vi "Base64ToHexString.vi"(1 "BASE64 string":string) -> (0 "Hex":string)   [LabVIEW 2023]
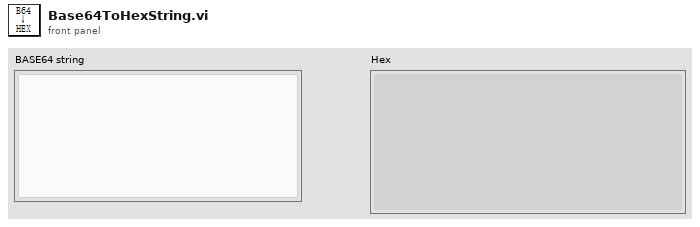
[diagram p1: front panel]
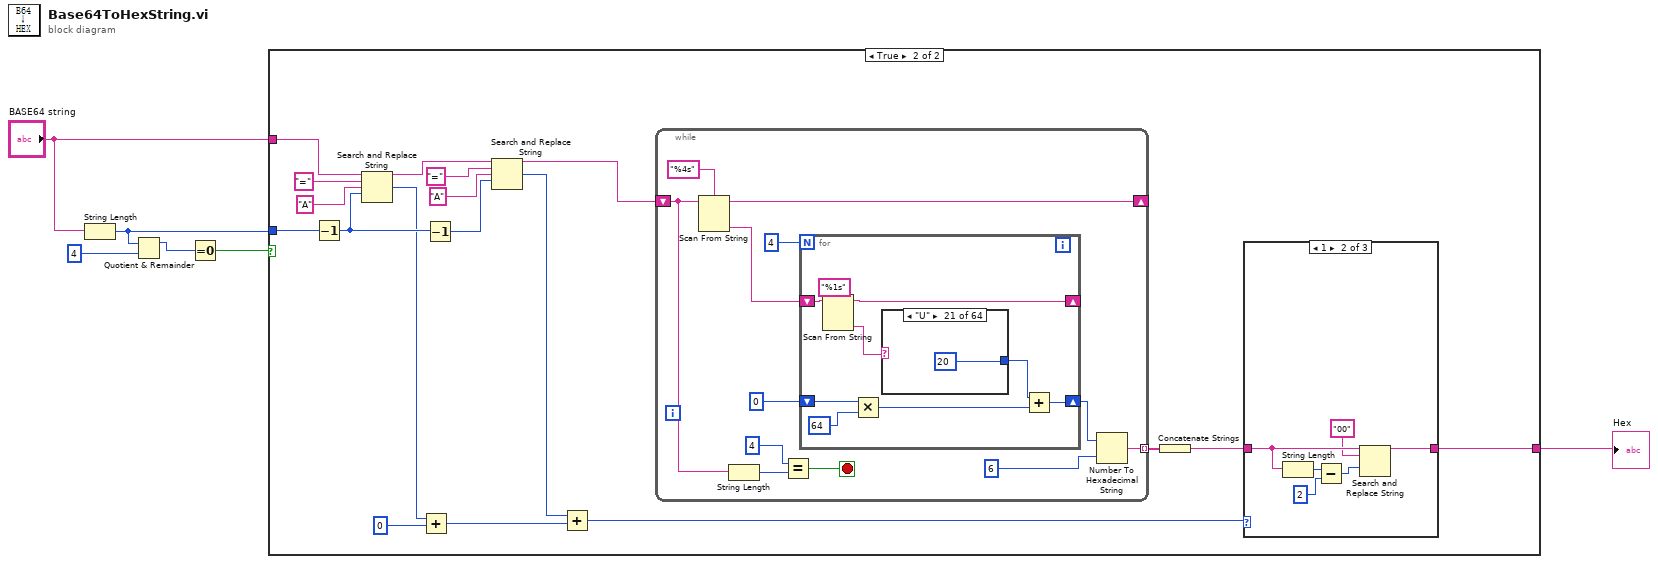
[diagram p0: block diagram]
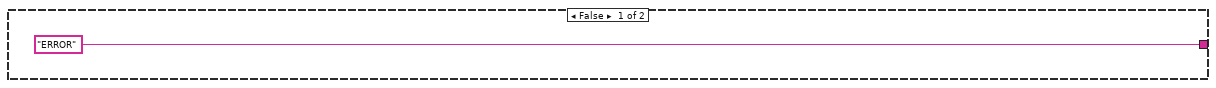
[diagram p2: hidden frame]
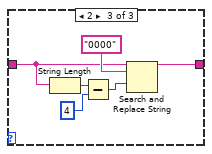
[diagram p4: hidden frame]
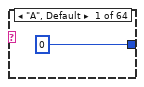
[diagram p5: hidden frame]
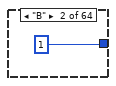
[diagram p6: hidden frame]
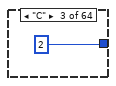
[diagram p7: hidden frame]
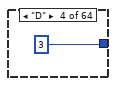
[diagram p8: hidden frame]
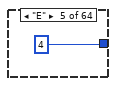
[diagram p9: hidden frame]
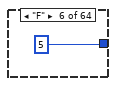
[diagram p10: hidden frame]
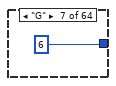
[diagram p11: hidden frame]
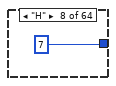
[diagram p12: hidden frame]
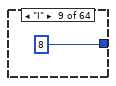
[diagram p13: hidden frame]
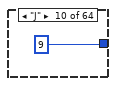
[diagram p14: hidden frame]
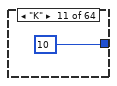
[diagram p15: hidden frame]
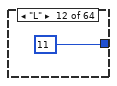
[diagram p16: hidden frame]
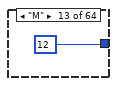
[diagram p17: hidden frame]
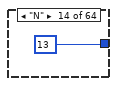
[diagram p18: hidden frame]
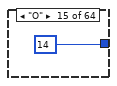
[diagram p19: hidden frame]
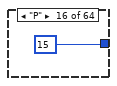
[diagram p20: hidden frame]
diagram:
  n1 = String Length(string="BASE64 string") -> (length=w4:i32)
  n2 = Quotient & Remainder(x=w4, y=4) -> (x-y*floor(x/y)=w3:i32)  [unwired: 1 out]
  n3 = Equal To 0?(x=w3) -> (x = 0?=w2:bool)
  n4 = case shown="True" w2 {
    tunnel: "BASE64 string" -> [_ w23]
    tunnel: w4 -> [_ w14]
    tunnel: ["ERROR" w8] -> w1
    frame False {
    }
    frame True {
      n5 = Decrement(x=w14) -> (x-1=w22:i32)
      n6 = Search and Replace String(input string=w23, search string="=", replace string="A", offset=w22) -> (result string=w19:string, number of replacements=w16:i32)  [unwired: 4 in, 2 out]
      n7 = Add(x=w16, y=0) -> (x+y=w17:i32)
      n8 = Decrement(x=w22) -> (x-1=w18:i32)
      n9 = Search and Replace String(input string=w19, search string="=", replace string="A", offset=w18) -> (result string=w12:string, number of replacements=w15:i32)  [unwired: 4 in, 2 out]
      n10 = Add(x=w15, y=w17) -> (x+y=w10:i32)
      n11 = while {
        shift-right: [w49] -> _
        shift-left: w12 -> [w41]
        tunnel: [w43] -> w11 mode=indexing
        stop <- w39 stop-if-true
        n12 = Scan From String(format string="%4s", input string=w41) -> (remaining string=w49:string, output 1=w48:string)  [unwired: 3 in, 2 out]
        n13 = String Length(string=w41) -> (length=w40:i32)
        n14 = Equal?(x=4, y=w40) -> (x = y?=w39:bool)
        n15 = for {
          N: 4 -> [_]
          shift-right: [w52] -> w45
          shift-left: 0 -> [w56]
          shift-right: [w51] -> _
          shift-left: w48 -> [w58]
          n16 = Scan From String(format string="%1s", input string=w58) -> (remaining string=w51:string, output 1=w57:string)  [unwired: 3 in, 2 out]
          n17 = Multiply(x=w56, y=64) -> (x*y=w54:i32)
          n18 = case shown="\"U\"" w57 {
            tunnel: [0 1 2 3 4 5 6 7 8 9 10 11 12 13 14 15 16 17 18 19 20 21 22 23 24 25 26 27 28 29 30 31 32 33 34 35 36 37 38 39 40 41 42 43 44 45 46 47 48 49 50 51 52 53 54 55 56 57 58 59 60 61 62 63] -> w53
            frame "A", Default {
            }
            frame "B" {
            }
            frame "C" {
            }
            frame "D" {
            }
            frame "E" {
            }
            frame "F" {
            }
            frame "G" {
            }
            frame "H" {
            }
            frame "I" {
            }
            frame "J" {
            }
            frame "K" {
            }
            frame "L" {
            }
            frame "M" {
            }
            frame "N" {
            }
            frame "O" {
            }
            frame "P" {
            }
            frame "Q" {
            }
            frame "R" {
            }
            frame "S" {
            }
            frame "T" {
            }
            frame "U" {
            }
            frame "V" {
            }
            frame "W" {
            }
            frame "X" {
            }
            frame "Y" {
            }
            frame "Z" {
            }
            frame "a" {
            }
            frame "b" {
            }
            frame "c" {
            }
            frame "d" {
            }
            frame "e" {
            }
            frame "f" {
            }
            frame "g" {
            }
            frame "h" {
            }
            frame "i" {
            }
            frame "j" {
            }
            frame "k" {
            }
            frame "l" {
            }
            frame "m" {
            }
            frame "n" {
            }
            frame "o" {
            }
            frame "p" {
            }
            frame "q" {
            }
            frame "r" {
            }
            frame "s" {
            }
            frame "t" {
            }
            frame "u" {
            }
            frame "v" {
            }
            frame "w" {
            }
            frame "x" {
            }
            frame "y" {
            }
            frame "z" {
            }
            frame "0" {
            }
            frame "1" {
            }
            frame "2" {
            }
            frame "3" {
            }
            frame "4" {
            }
            frame "5" {
            }
            frame "6" {
            }
            frame "7" {
            }
            frame "8" {
            }
            frame "9" {
            }
            frame "+" {
            }
            frame "/" {
            }
          }
          n19 = Add(x=w53, y=w54) -> (x+y=w52:i32)
        }
        n20 = Number To Hexadecimal String(1:6, 2:w45) -> (0:w43:string)
      }
      n21 = Concatenate Strings(w11) -> (w9:string)
      n22 = case shown="1" w10 {
        tunnel: [w26 w27 w34] -> w8
        tunnel: w9 -> [w26 w29 w33]
        frame 0, Default {
        }
        frame 1 {
          n23 = String Length(string=w29) -> (length=w31:i32)
          n24 = Subtract(x=w31, y=2) -> (x-y=w32:i32)
          n25 = Search and Replace String(input string=w29, search string="00", offset=w32) -> (result string=w27:string)  [unwired: 5 in, 3 out]
        }
        frame 2 {
          n26 = String Length(string=w33) -> (length=w37:i32)
          n27 = Subtract(x=w37, y=4) -> (x-y=w38:i32)
          n28 = Search and Replace String(input string=w33, search string="0000", offset=w38) -> (result string=w34:string)  [unwired: 5 in, 3 out]
        }
      }
    }
  }
  "Hex" <- w1
